vi "Set Configuration Cluster.vi"(10 "Framework Configuration":T1, 11 "Framework Configuration in":refnum<class "Framework Configuration.lvclass">) -> (3 "Framework Configuration out":refnum<class "Framework Configuration.lvclass">)   [LabVIEW 2017, in "Data Sharing Framework Core.lvlib" / "Data Sharing Framework Engine.lvlib" / "Framework Configuration.lvclass"]
uses:
  Framework Configuration.lvclass
  Configuration/1.0.0/Public/Controls/DSF Engine Framework Configuration.ctl
  Configuration/1.0.0/Public/Controls/DSF Engine Plugin Configuration.ctl
  Configuration/1.0.0/Public/Controls/DSF Timing Info.ctl
  Configuration/1.0.0/Public/Controls/DSF Engine Transfer Group Configuration.ctl
  Configuration/1.0.0/Public/Controls/DSF Direction.ctl
  Configuration/1.0.0/Public/Controls/DSF Engine Transfer Configuration.ctl
  Configuration/1.0.0/Public/Controls/DSF Byte Order.ctl
  Configuration/1.0.0/Public/Controls/DSF Engine Channel Configuration.ctl
  Configuration/1.0.0/Public/Controls/DSF Data Type.ctl
  Configuration/1.0.0/Public/Controls/DSF Settings Info.ctl
  Framework Configuration.lvclass/Framework Configuration.ctl
  Configuration/1.0.0/Data Sharing Framework Configuration.lvlib
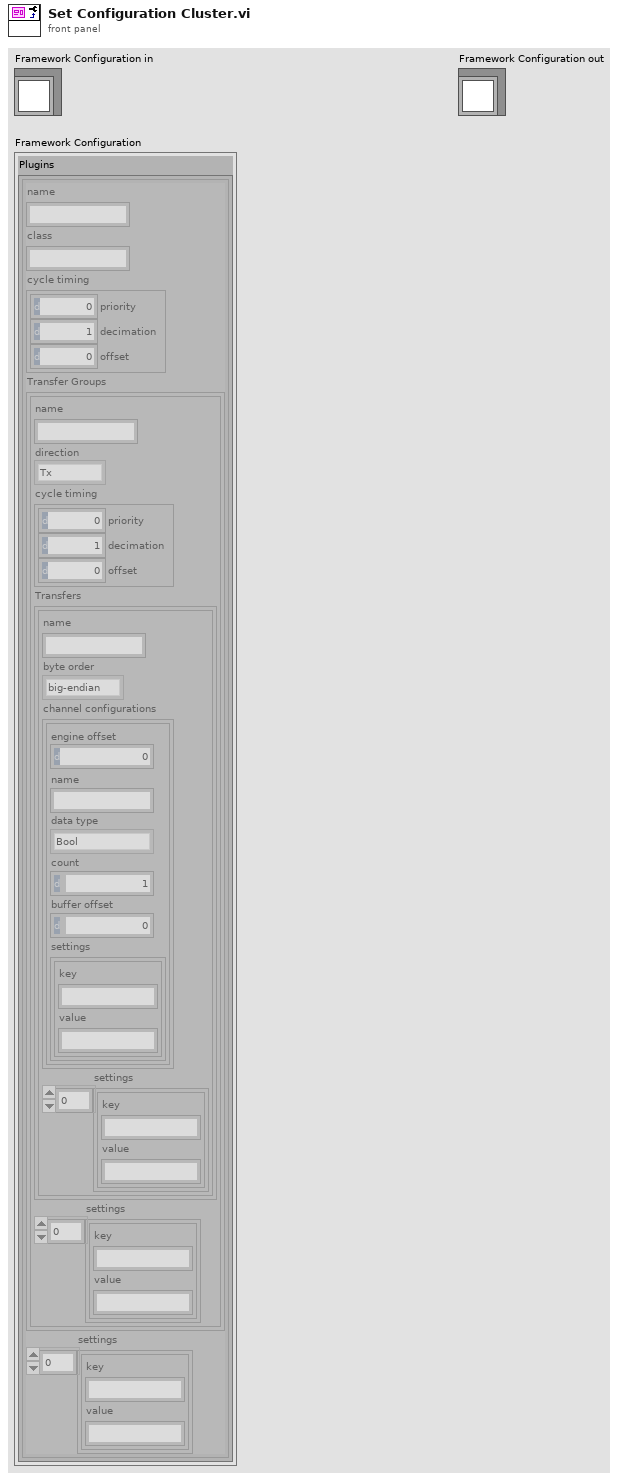
[diagram p1: front panel]
types:
  T1 = typedef "Data Sharing Framework Core.lvlib/Data Sharing Framework Configuration.lvlib/DSF Engine Framework Configuration.ctl" = cluster{"Plugins":T2[]}
  T2 = typedef "Data Sharing Framework Core.lvlib/Data Sharing Framework Configuration.lvlib/DSF Engine Plugin Configuration.ctl" = cluster{"name":string, "class":string, "cycle timing":T3, "Transfer Groups":T4[], "settings":T10}
  T3 = typedef "Data Sharing Framework Core.lvlib/Data Sharing Framework Configuration.lvlib/DSF Timing Info.ctl" = cluster{"priority":u64, "decimation":u64, "offset":u64}
  T4 = typedef "Data Sharing Framework Core.lvlib/Data Sharing Framework Configuration.lvlib/DSF Engine Transfer Group Configuration.ctl" = cluster{"name":string, "direction":T5, "cycle timing":T3, "Transfers":T6[], "settings":T10}
  T5 = typedef "Data Sharing Framework Core.lvlib/Data Sharing Framework Configuration.lvlib/DSF Direction.ctl" = enum8{"Tx", "Rx"}
  T6 = typedef "Data Sharing Framework Core.lvlib/Data Sharing Framework Configuration.lvlib/DSF Engine Transfer Configuration.ctl" = cluster{"name":string, "byte order":T7, "channel configurations":T8[], "settings":T10}
  T7 = typedef "Data Sharing Framework Core.lvlib/Data Sharing Framework Configuration.lvlib/DSF Byte Order.ctl" = enum8{"big-endian", "little-endian"}
  T8 = typedef "Data Sharing Framework Core.lvlib/Data Sharing Framework Configuration.lvlib/DSF Engine Channel Configuration.ctl" = cluster{"engine offset":u64, "name":string, "data type":T9, "count":u64, "buffer offset":u64, "settings":T10}
  T9 = typedef "Data Sharing Framework Core.lvlib/Data Sharing Framework Configuration.lvlib/DSF Data Type.ctl" = enum8{"Bool", "SGL", "DBL", "I8", "I16", "I32", "I64", "U8", "U16", "U32", "U64"}
  T10 = typedef "Data Sharing Framework Core.lvlib/Data Sharing Framework Configuration.lvlib/DSF Settings Info.ctl" = cluster{"key":string, "value":string}[]
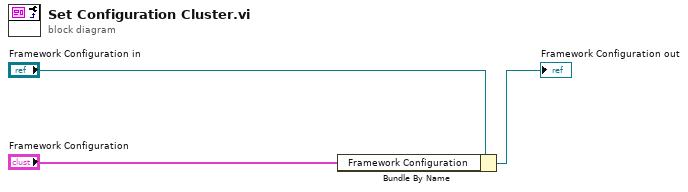
[diagram p0: block diagram]
diagram:
  n1 = Bundle By Name(cluster="Framework Configuration in", "Framework Configuration"="Framework Configuration") -> (→"Framework Configuration out":refnum<class "Framework Configuration.lvclass">)
